vi "Main2.vi"() -> ()   [LabVIEW 2014]
uses:
  Control/Control_process.ctl
  Program Files (x86)/National Instruments/LabVIEW 2018/instr.lib/OSICS 1.1.0/OSICS_LIB.lvlib
  <vilib>/Utility/file.llb/Write Delimited Spreadsheet (string).vi
panel:
  out "EXFO_OPC 2":bool
  out "EXFO_OPC":bool
  in  "myFname":bool caption="Naming Log"
  out "error IO":errorcluster
  out "Test_pts_array":dbl[](array[numeric])
  out "WL_now":dbl
  in  "stop":bool
  in  "WL_delay(ms)":u32=200
  in  "VISA_PWM":refnum<visa-resource-name> caption="Power Meter"
  in  "VISA_TLS":refnum<visa-resource-name> caption="Light Source"
  in  "PM_delay(ms)":i32=100
  out "Ref dbm":dbl caption="Ref (dBm)" format="%#.2g"
  in  "WL_Set":dbl=1310.0 caption="Wavelength"
  out "pow_read":dbl caption="Pow" format="%#.2g"
  in  "WL_step":dbl=1.0 caption="Step(nm)"
  out "WL_Peak":dbl caption="Peak"
  in  "WL_End":dbl=1350.0 caption="End(nm)"
  in  "WL_Start":dbl=1260.0 caption="Start(nm)"
  in  "Link Button":bool
  in  "Unit(dB:T)":bool
  in  "Read Button":bool
  in  "Ref Button":bool
  in  "Ref_spec Button":bool
  out "REF?":bool caption="Ref.1pt"
  out "testing?":bool caption="Busy"
  out "link?":bool caption="Online"
  out "Msg":string
  in  "Sweep Button":bool
  out "pow_chart":dbl(graph)
  # "切換波長有OPC?指令應該是會等待執行完成的flag回傳\n不須另外放delay, 目前有家只是為了確保"
  # "不紀錄取單點參考值的波長，全波長才記\n要考慮一下做了什麼動作就清掉全波長參考值"
  # "Equip."
  # "SWEEP"
  # "READ"
  # "Ver. B01.0"
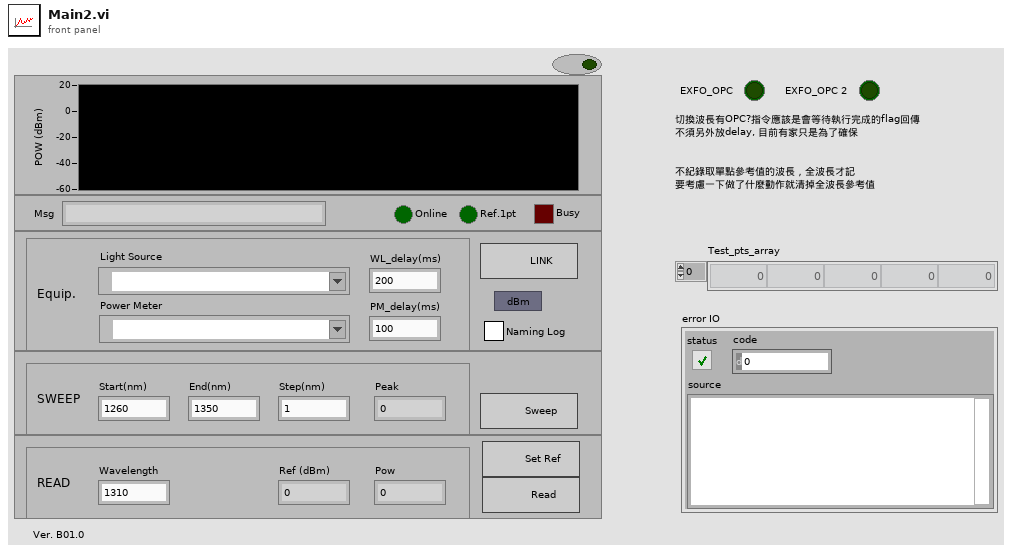
[diagram p1: front panel]
types:
  T1 = typedef "Control_process.ctl" = enum16{"init", "link", "reference", "reference2", "wave_chng", "lockpanel", "single", "sweep", "log_res", "quit"}
  T2 = enum8{"Enabled", "Disabled", "Disabled and Grayed Out"}
  T3 = cluster{"Laser State":bool, "WL/F Value":dbl, "Power (dBm/mW)":dbl, "Power Limit":bool}
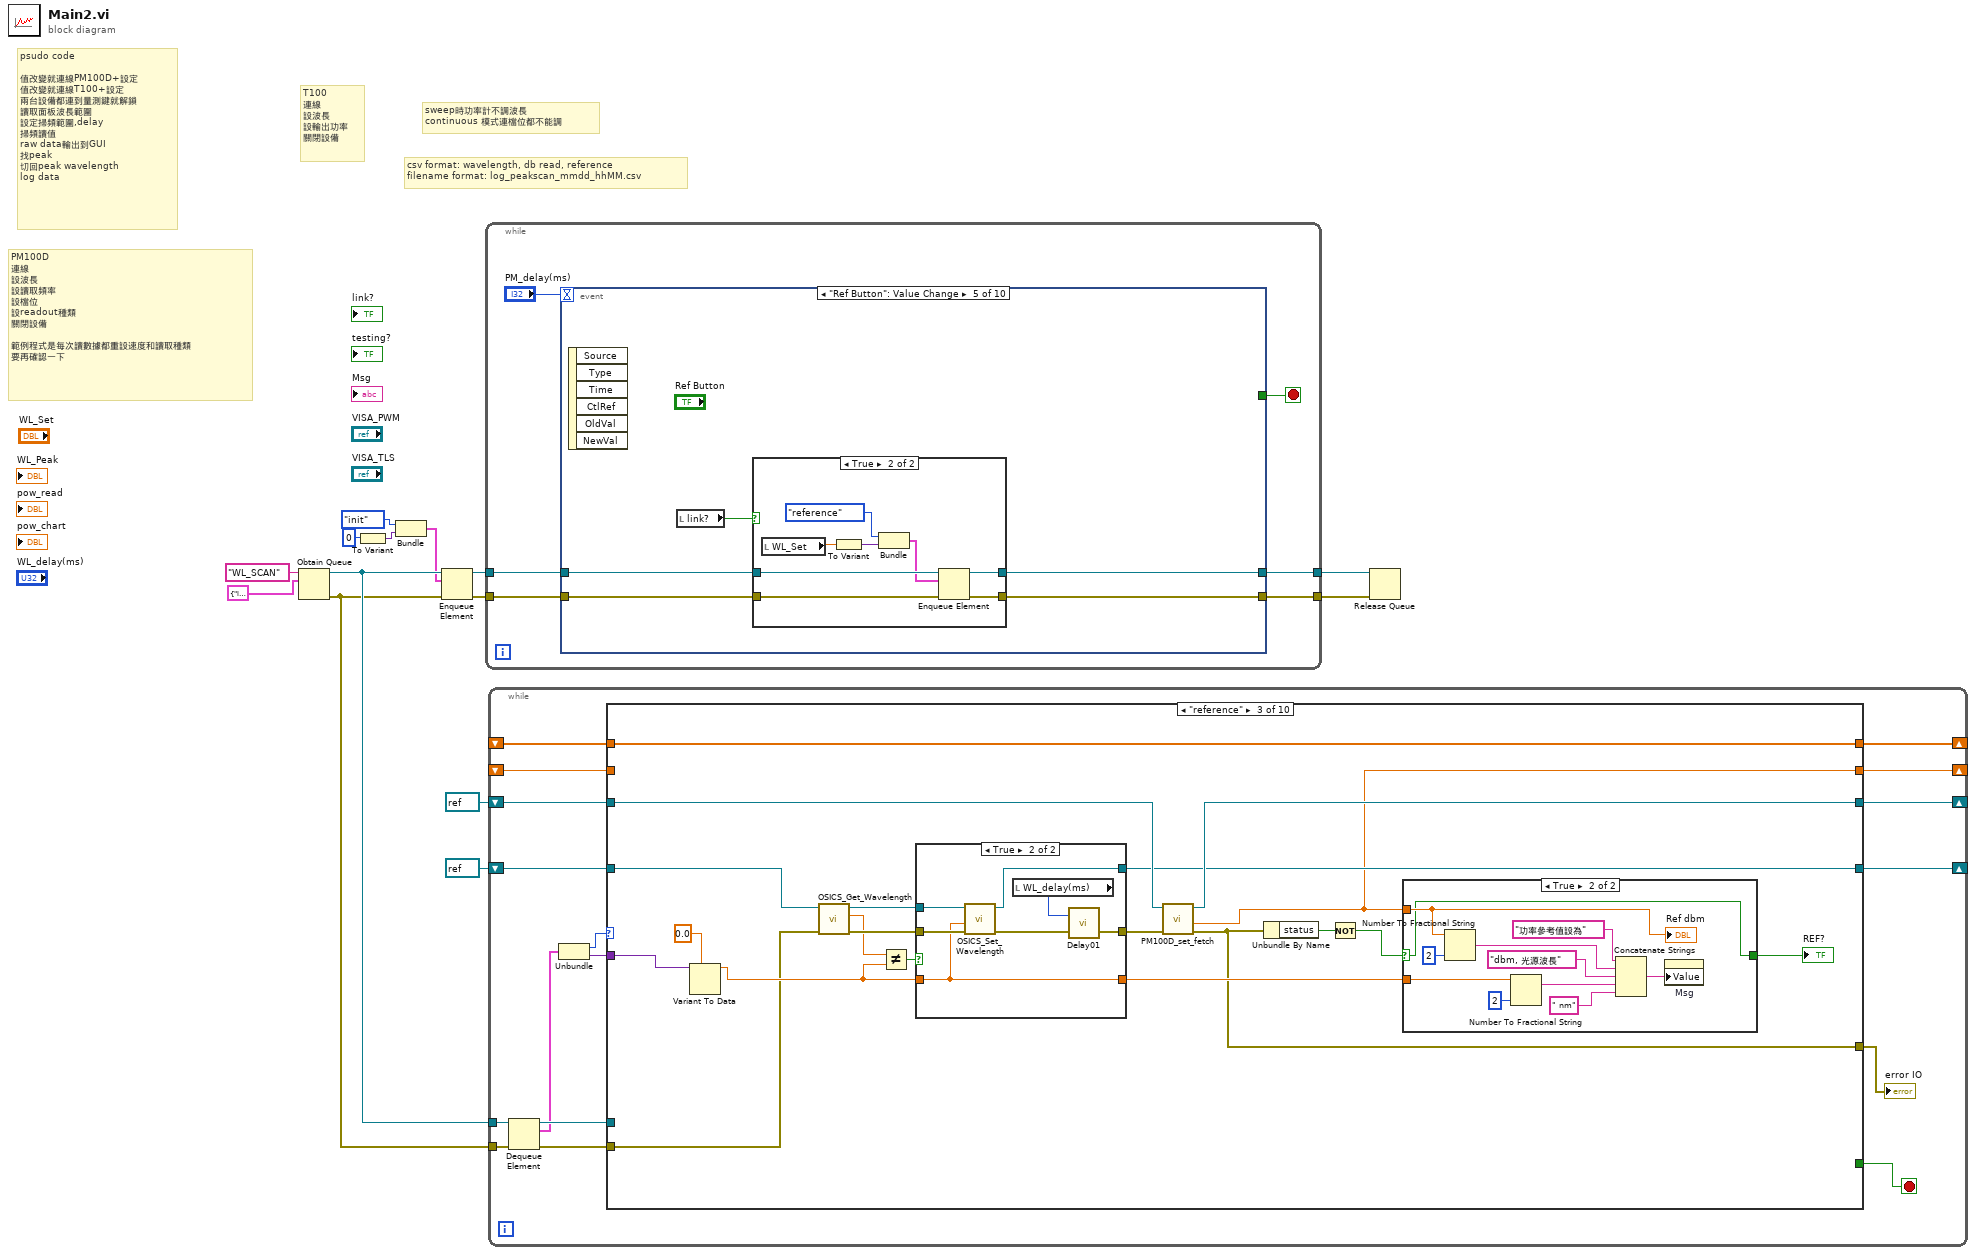
[diagram p0: block diagram]
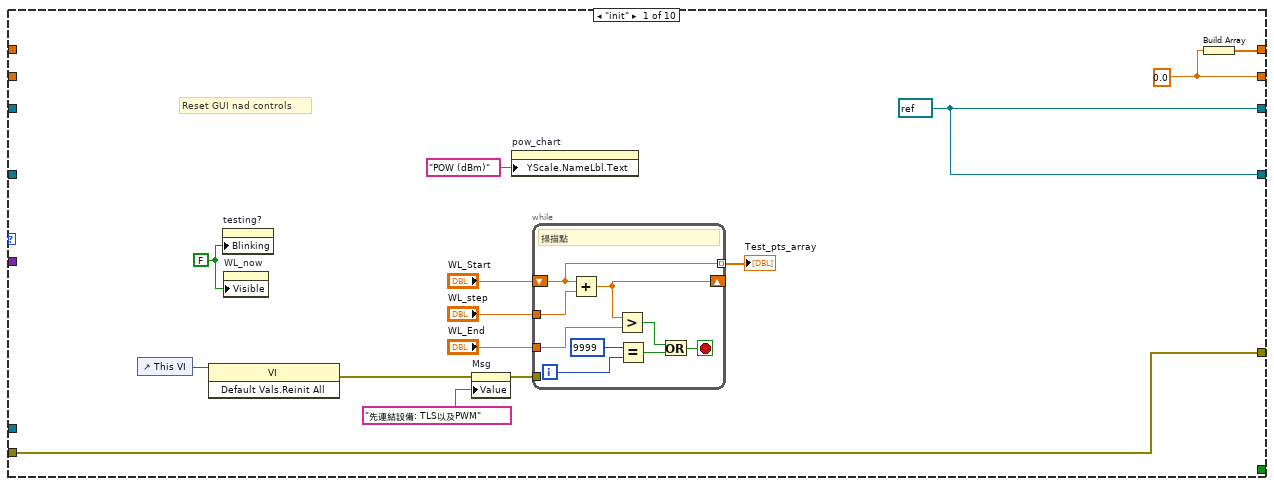
[diagram p2: hidden frame]
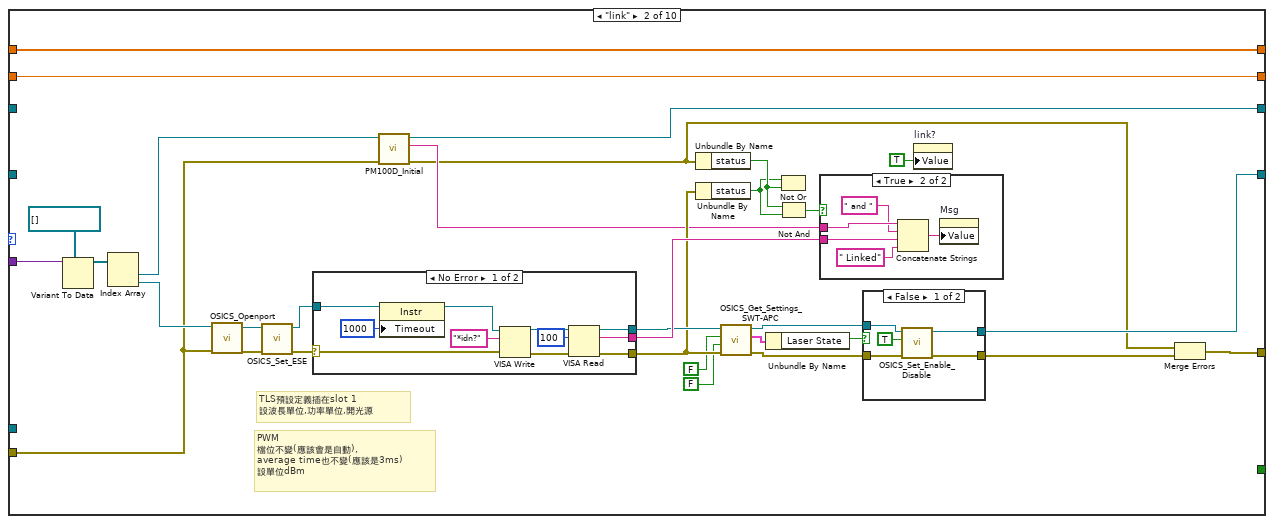
[diagram p3: hidden frame]
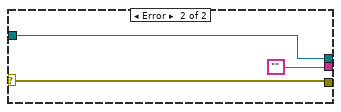
[diagram p4: hidden frame]
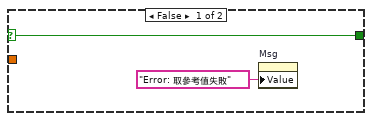
[diagram p7: hidden frame]
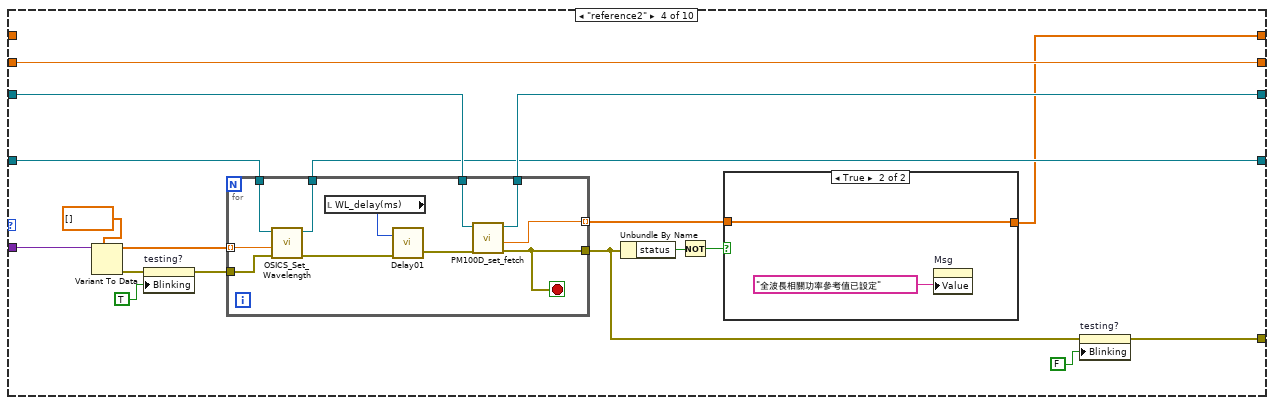
[diagram p9: hidden frame]
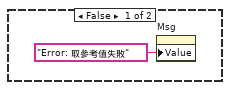
[diagram p10: hidden frame]
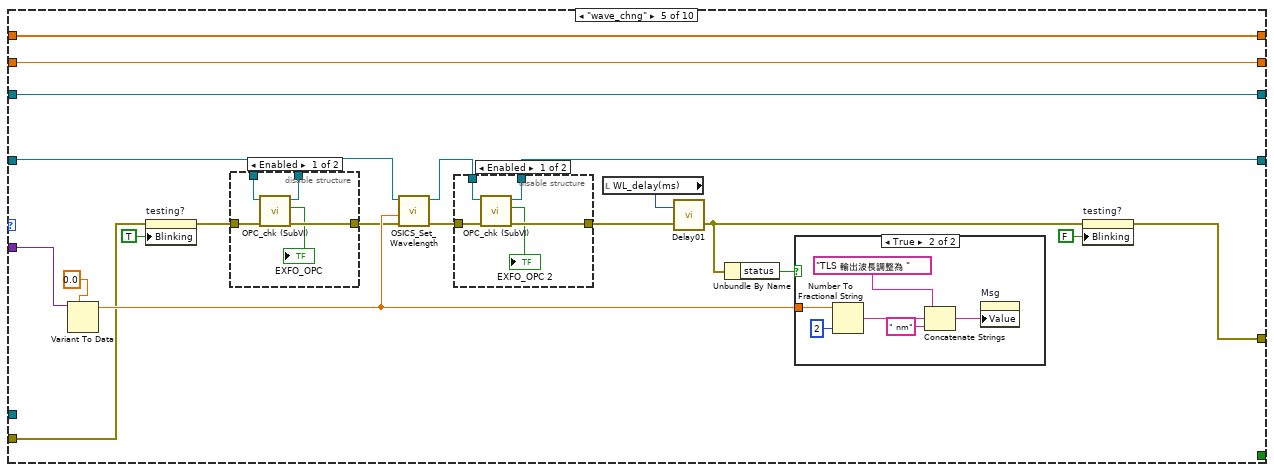
[diagram p11: hidden frame]
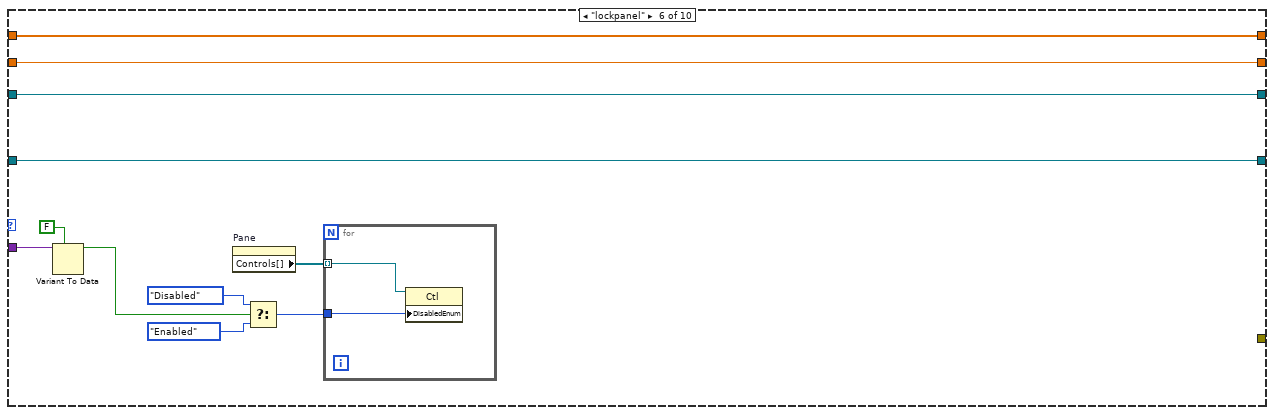
[diagram p15: hidden frame]
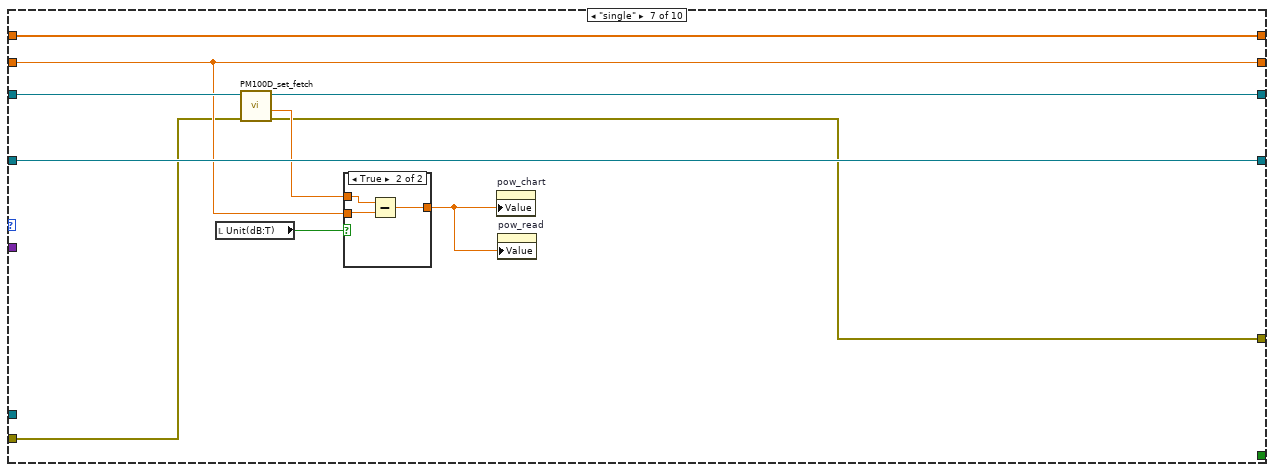
[diagram p16: hidden frame]
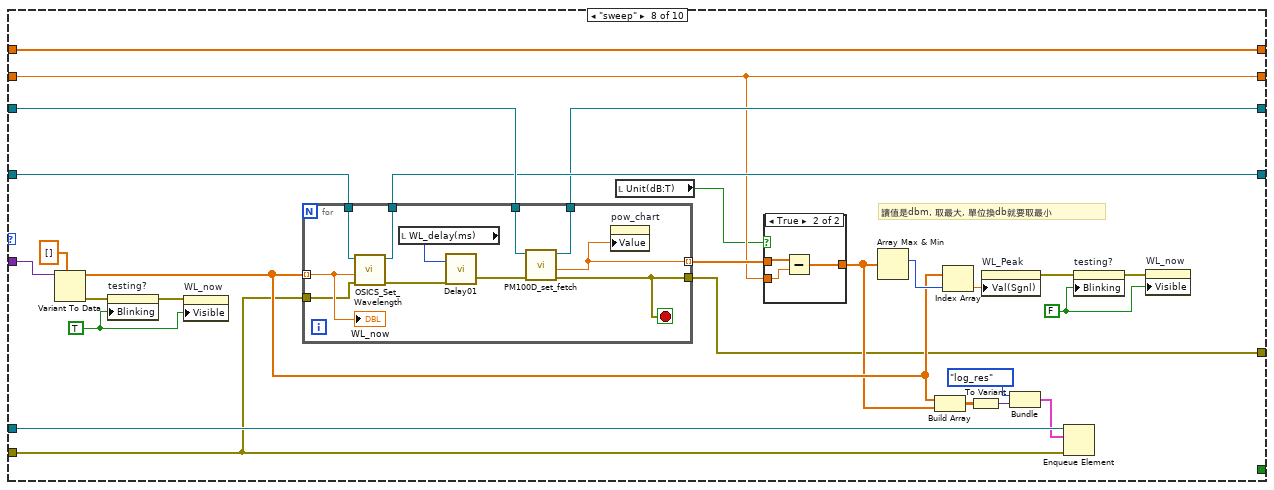
[diagram p18: hidden frame]
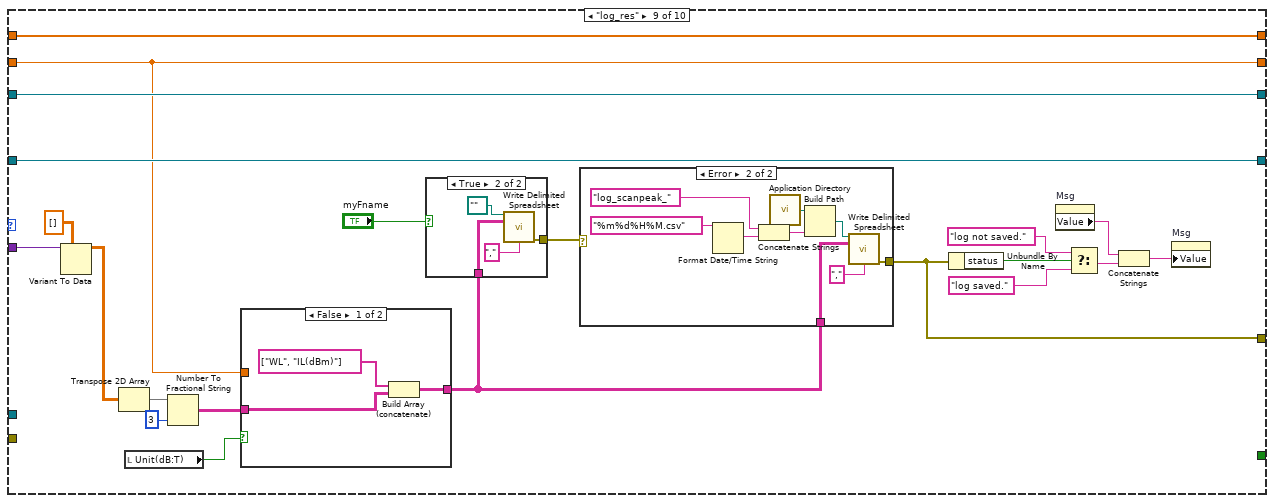
[diagram p20: hidden frame]
diagram:
  # "csv format: wavelength, db read, reference\nfilename format: log_peakscan_mmdd_hhMM.csv"
  # "sweep時功率計不調波長\ncontinuous 模式連檔位都不能調"
  # "T100\n連線\n設波長\n設輸出功率\n關閉設備"
  # "PM100D\n連線\n設波長\n設讀取頻率\n設檔位\n設readout種類\n關閉設備\n\n範例程式是每次讀數據都重設速度和讀取種類\n要再確認一下"
  # "psudo code\n\n值改變就連線PM100D+設定\n值改變就連線T100+設定\n兩台設備都連到量測鍵就解鎖\n讀取面板波長範圍\n設定掃頻範圍,delay\n掃頻讀值\nraw data輸出到GUI\n找peak\n切回peak wavelength\nlog data"
  n1 = Obtain Queue(name (unnamed)="WL_SCAN", element data type=cluster{"Proc":T1, variant} {"Proc"=enum."init", variant}) -> (queue out=w13:refnum<queue>, error out=w1:errorcluster)  [unwired: 3 in, 1 out]
  n2 = To Variant(anything=0) -> (Variant=w6:variant)
  n3 = Bundle("Proc"=Control_process."init", "Variant"=w6) -> (w4:cluster{"Proc":T1, "Variant":variant})  [unwired: 1 in]
  n4 = Enqueue Element(queue=w13, element=w4, error in (no error)=w1) -> (queue out=w9:refnum<queue>, error out=w8:errorcluster)  [unwired: 1 in, 1 out]
  n5 = while {
    tunnel: w9 -> [w18]
    tunnel: w8 -> [w19]
    tunnel: [w17] -> w12
    tunnel: [w16] -> w11
    stop <- w20 stop-if-true
    n6 = event shown="[4] \"Ref Button\": Value Change" {
      selector: _ -> [_ _ _ _ _ _ _ _ _ _]
      dyn-events: _ -> [_ _ _ _ _ _ _ _ _ _]
      timeout: "PM_delay(ms)" -> [_ _ _ _ _ _ _ _ _ _]
      tunnel: [_ _ _ _ _ _ _ _ _ TRUE] -> w20
      tunnel: w19 -> [w26 w40 w53 w75 w89 w105 w136 w146 w174 w196]
      tunnel: w18 -> [w27 w41 w54 w76 w90 w106 w132 w148 w177 w194]
      tunnel: [w25 w41 w52 w76 w88 w104 w131 w147 w176 w193] -> w17
      tunnel: [w24 w40 w51 w75 w87 w103 w136 w145 w175 w195] -> w16
      event Timeout {
        n7 = event-data() -> ()  [unwired: 1 in, 3 out]
        n8 = local read "link?"() -> (w21:bool)
        n9 = local read "Read Button"() -> (w22:bool)
        n10 = And(x=w21, y=w22) -> (x .and. y?=w23:bool)
        n11 = case shown="False" w23 {
          tunnel: w27 -> [w29 w37]
          tunnel: w26 -> [w28 w36]
          tunnel: [w29 w35] -> w25
          tunnel: [w28 w34] -> w24
          frame False {
          }
          frame True {
            n12 = To Variant(anything=0) -> (Variant=w33:variant)
            n13 = Bundle("Proc"=Control_process."single", "Variant"=w33) -> (w31:cluster{"Proc":T1, "Variant":variant})  [unwired: 1 in]
            n14 = Enqueue Element(queue=w37, element=w31, error in (no error)=w36) -> (queue out=w35:refnum<queue>, error out=w34:errorcluster)  [unwired: 1 in, 1 out]
          }
        }
      }
      event "Unit(dB:T)": Value Change {
        # "這個事件會卡有紀錄參考值才能把單位轉dB"
        n15 = event-data() -> ()  [unwired: 1 in, 6 out]
        n16 = local read "REF?"() -> (w39:bool)
        n17 = case shown="True" w39 {
          tunnel: "Unit(dB:T)" -> [_ w47]
          frame False {
            n18 = property on="Unit(dB:T)" class="Bool (strict)"("Value"=FALSE ("Unit")) -> ()  [unwired: 2 in, 2 out]
            n19 = property on="Msg" class="Str"("Value"="Error: 參考值未設定" ("Msg")) -> ()  [unwired: 2 in, 2 out]
          }
          frame True {
            n20 = Select(t="POW (dB)", s=w47, f="POW (dBm)") -> (s? t:f=w48:string)
            n21 = property on="pow_chart" class="WFChart (strict)"("YScale.NameLbl.Text"=w48, "History Data"=dbl[] []) -> ()  [unwired: 2 in, 2 out]
          }
        }
      }
      event "Link Button": Value Change {
        n22 = event-data() -> ()  [unwired: 1 in, 1 out]
        n23 = local read "VISA_PWM"() -> (w49:refnum<visa-resource-name>)
        n24 = local read "VISA_TLS"() -> (w50:refnum<visa-resource-name>)
        n25 = Empty String/Path?(string/path=w50) -> (empty?=w56:bool)
        n26 = Empty String/Path?(string/path=w49) -> (empty?=w57:bool)
        n27 = Not Or(1:w56, 2:w57) -> (0:w55:bool)
        n28 = case shown="True" w55 {
          tunnel: w54 -> [w60 w70]
          tunnel: w53 -> [w59 w69]
          tunnel: [w60 w68] -> w52
          tunnel: [w59 w67] -> w51
          tunnel: w49 -> [_ w64]
          tunnel: w50 -> [_ w63]
          frame False {
            n29 = property on="Msg" class="Str"("Value"="Error: 未選擇儀器位址" ("Msg")) -> ()  [unwired: 2 in, 2 out]
          }
          frame True {
            n30 = Build Array(w64, w63) -> (w62:refnum<visa-resource-name>[])
            n31 = To Variant(anything=w62) -> (Variant=w61:variant)
            n32 = Bundle("Proc"=Control_process."link", "Variant"=w61) -> (w65:cluster{"Proc":T1, "Variant":variant})  [unwired: 1 in]
            n33 = Enqueue Element(queue=w70, element=w65, error in (no error)=w69) -> (queue out=w68:refnum<queue>, error out=w67:errorcluster)  [unwired: 1 in, 1 out]
          }
        }
      }
      event "WL_Start", "WL_End", "WL_step": Value Change {
        n34 = event-data() -> ()  [unwired: 1 in, 6 out]
        n35 = local read "WL_Start"() -> (w72:dbl)
        n36 = local read "WL_step"() -> (w74:dbl)
        n37 = local read "WL_End"() -> (w73:dbl)
        n38 = while {
          tunnel: w74 -> [w80]
          tunnel: w73 -> [w79]
          shift-right: [w81] -> _
          shift-left: w72 -> [w82]
          tunnel: [w82] -> w71 mode=indexing
          i -> [w78]
          stop <- w77 stop-if-true
          # "掃描點"
          n39 = Add(x=w82, y=w80) -> (x+y=w81:dbl)
          n40 = Greater?(x=w81, y=w79) -> (0:w84:bool)
          n41 = Equal?(x=9999, y=w78) -> (x = y?=w83:bool)
          n42 = Or(x=w84, y=w83) -> (x .or. y?=w77:bool)
        }
        n43 = local write "Test_pts_array"(w71) -> ()
      }
      event "Ref Button": Value Change {
        n44 = event-data() -> ()  [unwired: 1 in, 6 out]
        n45 = local read "link?"() -> (w86:bool)
        n46 = case shown="True" w86 {
          tunnel: w90 -> [w93 w101]
          tunnel: w89 -> [w92 w100]
          tunnel: [w93 w99] -> w88
          tunnel: [w92 w98] -> w87
          frame False {
            n47 = property on="Msg" class="Str"("Value"="Err: 設備未連結" ("Msg")) -> ()  [unwired: 2 in, 2 out]
          }
          frame True {
            n48 = local read "WL_Set"() -> (w94:dbl)
            n49 = To Variant(anything=w94) -> (Variant=w97:variant)
            n50 = Bundle("Proc"=Control_process."reference", "Variant"=w97) -> (w95:cluster{"Proc":T1, "Variant":variant})  [unwired: 1 in]
            n51 = Enqueue Element(queue=w101, element=w95, error in (no error)=w100) -> (queue out=w99:refnum<queue>, error out=w98:errorcluster)  [unwired: 1 in, 1 out]
          }
        }
      }
      event "Ref_spec Button": Value Change {
        n52 = event-data() -> ()  [unwired: 1 in, 6 out]
        n53 = local read "link?"() -> (w102:bool)
        n54 = case shown="True" w102 {
          tunnel: w106 -> [w109 w117]
          tunnel: w105 -> [w108 w116]
          tunnel: [w109 w113] -> w104
          tunnel: [w108 w110] -> w103
          frame False {
            n55 = property on="Msg" class="Str"("Value"="Error: 設備未連結" ("Msg")) -> ()  [unwired: 2 in, 2 out]
          }
          frame True {
            n56 = To Variant(anything=TRUE) -> (Variant=w123:variant)
            n57 = Bundle("Proc"=Control_process."lockpanel", "Variant"=w123) -> (w125:cluster{"Proc":T1, "Variant":variant})  [unwired: 1 in]
            n58 = local read "WL_Set"() -> (w126:dbl)
            n59 = Enqueue Element(queue=w117, element=w125, error in (no error)=w116) -> (queue out=w111:refnum<queue>, error out=w115:errorcluster)  [unwired: 1 in, 1 out]
            n60 = To Variant(anything=w126) -> (Variant=w129:variant)
            n61 = Bundle("Proc"=Control_process."reference", "Variant"=w129) -> (w127:cluster{"Proc":T1, "Variant":variant})  [unwired: 1 in]
            n62 = Enqueue Element(queue=w111, element=w127, error in (no error)=w115) -> (queue out=w112:refnum<queue>, error out=w114:errorcluster)  [unwired: 1 in, 1 out]
            n63 = To Variant(anything=FALSE) -> (Variant=w120:variant)
            n64 = Bundle("Proc"=Control_process."lockpanel", "Variant"=w120) -> (w118:cluster{"Proc":T1, "Variant":variant})  [unwired: 1 in]
            n65 = Enqueue Element(queue=w112, element=w118, error in (no error)=w114) -> (queue out=w113:refnum<queue>, error out=w110:errorcluster)  [unwired: 1 in, 1 out]
          }
        }
      }
      event "Read Button": Value Change {
        n66 = event-data() -> ()  [unwired: 1 in, 6 out]
        n67 = local read "link?"() -> (w134:bool)
        n68 = And(x=w134, y="Read Button") -> (x .and. y?=w133:bool)
        n69 = case shown="False" w133 {
          selector: w133 -> [w141 w142]
          tunnel: w132 -> [w139 w143]
          tunnel: [w138 w143] -> w131
          tunnel: [FALSE ("Blinking") w142] -> w130
          frame False {
            n70 = property on="Read Button" class="Bool (strict)"("Value"=w141) -> ()  [unwired: 2 in, 2 out]
            n71 = property on="Msg" class="Str"("Value"="Error: 設備未連結" ("Msg")) -> ()  [unwired: 2 in, 2 out]
            n72 = Flush Queue(queue=w139) -> (queue out=w138:refnum<queue>)  [unwired: 1 in, 2 out]
          }
          frame True {
          }
        }
        n73 = property on="testing?" class="Bool (strict)"("Blinking"=w130) -> ()  [unwired: 2 in, 2 out]
      }
      event "Sweep Button": Value Change {
        n74 = event-data() -> ()  [unwired: 1 in, 1 out]
        n75 = local read "link?"() -> (w144:bool)
        n76 = case shown="True" w144 {
          tunnel: w148 -> [w151 w155]
          tunnel: [w151 w161] -> w147
          tunnel: w146 -> [w150 w159]
          tunnel: [w150 w156] -> w145
          frame False {
            n77 = property on="Msg" class="Str"("Value"="Err: 設備未連結" ("Msg")) -> ()  [unwired: 2 in, 2 out]
          }
          frame True {
            n78 = To Variant(anything=TRUE) -> (Variant=w167:variant)
            n79 = Bundle("Proc"=Control_process."lockpanel", "Variant"=w167) -> (w168:cluster{"Proc":T1, "Variant":variant})  [unwired: 1 in]
            n80 = local read "Test_pts_array"() -> (w152:dbl[])
            n81 = Enqueue Element(queue=w155, element=w168, error in (no error)=w159) -> (queue out=w154:refnum<queue>, error out=w158:errorcluster)  [unwired: 1 in, 1 out]
            n82 = To Variant(anything=w152) -> (Variant=w171:variant)
            n83 = Bundle("Proc"=Control_process."sweep", "Variant"=w171) -> (w170:cluster{"Proc":T1, "Variant":variant})  [unwired: 1 in]
            n84 = Enqueue Element(queue=w154, element=w170, error in (no error)=w158) -> (queue out=w153:refnum<queue>, error out=w157:errorcluster)  [unwired: 1 in, 1 out]
            n85 = To Variant(anything=FALSE) -> (Variant=w164:variant)
            n86 = Bundle("Proc"=Control_process."lockpanel", "Variant"=w164) -> (w163:cluster{"Proc":T1, "Variant":variant})  [unwired: 1 in]
            n87 = Enqueue Element(queue=w153, element=w163, error in (no error)=w157) -> (queue out=w161:refnum<queue>, error out=w156:errorcluster)  [unwired: 1 in, 1 out]
            n88 = property on="Msg" class="Str"("Value"="波長掃描中......" ("Msg")) -> ()  [unwired: 2 in, 2 out]
          }
        }
      }
      event "WL_Set", "WL_Peak": Value Change {
        n89 = event-data() -> ("NewVal"=w178:dbl)  [unwired: 1 in]
        n90 = local read "link?"() -> (w173:bool)
        n91 = case shown="True" w173 {
          tunnel: w178 -> [_ w187]
          tunnel: w177 -> [w180 w185]
          tunnel: [w180 w184] -> w176
          tunnel: [w179 w183] -> w175
          tunnel: w174 -> [w179 w182]
          frame False {
          }
          frame True {
            n92 = To Variant(anything=w187) -> (Variant=w188:variant)
            n93 = Bundle("Proc"=Control_process."wave_chng", "Variant"=w188) -> (w181:cluster{"Proc":T1, "Variant":variant})  [unwired: 1 in]
            n94 = Enqueue Element(queue=w185, element=w181, error in (no error)=w182) -> (queue out=w184:refnum<queue>, error out=w183:errorcluster)  [unwired: 1 in, 1 out]
          }
        }
      }
      event "stop": Value Change {
        n95 = event-data() -> ()  [unwired: 1 in, 6 out]
        n96 = local read "link?"() -> (w189:bool)
        n97 = To Variant(anything=w189) -> (Variant=w191:variant)
        n98 = Bundle("Proc"=Control_process."quit", "Variant"=w191) -> (w190:cluster{"Proc":T1, "Variant":variant})  [unwired: 1 in]
        n99 = Enqueue Element At Opposite End(queue=w194, element=w190, error in (no error)=w196) -> (queue out=w193:refnum<queue>, error out=w195:errorcluster)  [unwired: 1 in, 1 out]
      }
    }
  }
  n100 = while {
    tunnel: w13 -> [w214]
    shift-right: [w204] -> _
    shift-left: refnum<visa-resource-name> refnum ("instrument handle out") -> [w208]
    shift-right: [w207] -> _
    shift-left: refnum<visa-resource-name> refnum ("VISA OUT") -> [w206]
    shift-right: [w203] -> _
    shift-left: _ -> [w202]
    tunnel: w1 -> [w200]
    shift-right: [w198] -> _
    shift-left: _ -> [w199]
    stop <- w205 stop-if-true
    n101 = Dequeue Element(queue=w214, error in (no error)=w200) -> (queue out=w213:refnum<queue>, element=w211:cluster{"Proc":T1, variant}, error out=w212:errorcluster)  [unwired: 1 in, 1 out]
    n102 = Unbundle(w211) -> ("Proc"=w210:T1, w209:variant)
    n103 = case shown="\"reference\"" w210 {
      tunnel: w213 -> [_ _ _ _ _ _ _ w456 _ _]
      tunnel: w212 -> [w226 w239 w302 _ w379 _ w425 w439 _ w529]
      tunnel: w209 -> [_ w268 w312 w355 w390 w414 _ w463 w499 w533]
      tunnel: w208 -> [_ _ w314 w350 w386 w420 w433 w464 w491 w536]
      tunnel: [w228 w252 w311 w348 w372 w419 w432 w462 w498 w534] -> w207
      tunnel: w206 -> [_ _ w309 w351 w374 w419 w432 w461 w498 w538]
      tunnel: [_ _ _ _ _ _ _ _ _ TRUE] -> w205
      tunnel: [w228 w244 w313 w349 w386 w420 w431 w451 w491 w535] -> w204
      tunnel: [w226 w248 w301 w344 w382 _ w426 w446 w486 w528] -> w201
      tunnel: [w219 w249 w298 w352 w384 w421 w429 w449 w485 w530] -> w203
      tunnel: w202 -> [_ w249 _ w352 w384 w421 w429 w449 w485 w530]
      tunnel: w199 -> [_ w238 w295 _ w370 w411 w424 w438 w480 w526]
      tunnel: [w218 w238 w295 w339 w370 w411 w424 w438 w480 w526] -> w198
      frame "init" {
        w219 = 0.0
        w225 = FALSE ("Blinking")
        w228 = refnum<visa-resource-name> refnum ("instrument handle out")
        # "Reset GUI nad controls"
        n104 = control-ref of="This VI"() -> (w227:refnum<vi>)
        n105 = invoke class="VI" method="Default Vals.Reinit All"(reference=w227) -> (error out=w216:errorcluster)  [unwired: 2 in, 2 out]
        n106 = property on="testing?" class="Bool (strict)"("Blinking"=w225) -> ()  [unwired: 2 in, 2 out]
        n107 = property on="WL_now" class="DigNum (strict)"("Visible"=w225) -> ()  [unwired: 2 in, 2 out]
        n108 = property on="Msg" class="Str"(error in=w216, "Value"="先連結設備: TLS以及PWM" ("string")) -> (error out=w215:errorcluster)  [unwired: 1 in, 1 out]
        n109 = property on="pow_chart" class="WFChart (strict)"("YScale.NameLbl.Text"="POW (dBm)") -> ()  [unwired: 2 in, 2 out]
        n110 = while {
          tunnel: "WL_step" -> [w232]
          tunnel: "WL_End" -> [w231]
          shift-right: [w233] -> _
          shift-left: "WL_Start" -> [w234]
          tunnel: [w234] -> w221 mode=indexing
          tunnel: w215 -> [_]
          i -> [w230]
          stop <- w229 stop-if-true
          # "掃描點"
          n111 = Add(x=w234, y=w232) -> (x+y=w233:dbl)
          n112 = Greater?(x=w233, y=w231) -> (0:w236:bool)
          n113 = Equal?(x=9999, y=w230) -> (x = y?=w235:bool)
          n114 = Or(x=w236, y=w235) -> (x .or. y?=w229:bool)
        }
        "Test_pts_array" <- w221
        n115 = Build Array(w219) -> (w218:dbl[])
      }
      frame "link" {
        # "TLS預設定義插在slot 1\n設波長單位,功率單位,開光源"
        # "PWM\n檔位不變(應該會是自動), \naverage time也不變(應該是3ms)\n設單位dBm"
        n116 = Variant To Data(type=refnum<visa-resource-name>[] [], Variant=w268) -> (data=w267:refnum<visa-resource-name>[])  [unwired: 1 in, 1 out]
        n117 = Index Array(array=w267) -> (element #1=w245:refnum<visa-resource-name>, element #2=w265:refnum<visa-resource-name>)  [unwired: 2 in]
        n118 = call "OSICS_Openport.vi"("error in"=w239, "VISA IN"=w265) -> ("error out"=w266:errorcluster, "VISA OUT"=w264:refnum<visa-resource-name>)  [unwired: 8 in]
        n119 = call "OSICS_Set_ESE.vi"("error in (no error)"=w266, "VISA resource name"=w264) -> ("error out"=w242:errorcluster, "VISA resource name out"=w263:refnum<visa-resource-name>)  [unwired: 8 in]
        n120 = case shown="No Error" w242 {
          selector: w242 -> [w269 w282]
          tunnel: w263 -> [w273 w281]
          tunnel: [w272 ""] -> w262
          tunnel: [w271 w281] -> w260
          tunnel: [w270 w282] -> w257
          frame No Error {
            n121 = property class="Instr"(reference=w273, "Timeout"=u32 1000 ("General Settings:Timeout Value")) -> (reference out=w278:refnum<visa-resource-name>)  [unwired: 1 in, 1 out]
            n122 = VISA Write(VISA resource name=w278, write buffer="*idn?", error in (no error)=w269) -> (VISA resource name out=w276:refnum<visa-resource-name>, error out=w274:errorcluster)  [unwired: 1 out]
            n123 = VISA Read(VISA resource name=w276, byte count=u32 100, error in (no error)=w274) -> (VISA resource name out=w271:refnum<visa-resource-name>, read buffer=w272:string, error out=w270:errorcluster)  [unwired: 1 out]
          }
          frame Error {
          }
        }
        n124 = call "PM100D_Initial.vi"("error in"=w239, "VISA in"=w245) -> ("error out"=w243:errorcluster, "IDN String"=w246:string, "VISA out"=w244:refnum<visa-resource-name>)  [unwired: 2 in, 1 out]
        n125 = Unbundle By Name(w243) -> ("status"=w251:bool)
        n126 = Unbundle By Name(w257) -> ("status"=w250:bool)
        n127 = call "OSICS_Get_Settings_SWT-APC.vi"("error in"=w257, "Power Unit(dBm/mW)"=FALSE, "WL/F unit (nm/GHz)"=FALSE, "VISA IN"=w260) -> ("error out"=w253:errorcluster, "Laser Settings (Cluster)"=w259:T3, "VISA OUT"=w254:refnum<visa-resource-name>)  [unwired: 5 in]
        n128 = Unbundle By Name(w259) -> ("Laser State"=w258:bool)
        n129 = Not Or(1:w251, 2:w250) -> ()  [unwired: 1 out]
        n130 = Not And(1:w250, 2:w251) -> (0:w261:bool)
        n131 = case shown="True" w261 {
          tunnel: w262 -> [_ w294]
          tunnel: w246 -> [_ w293]
          frame False {
          }
          frame True {
            n132 = Concatenate Strings(w293, " and " ("string"), w294, " Linked" ("string")) -> (w291:string)
            n133 = property on="Msg" class="Str"("Value"=w291) -> ()  [unwired: 2 in, 2 out]
          }
        }
        n134 = case shown="False" w258 {
          tunnel: w254 -> [w286 w289]
          tunnel: w253 -> [w285 w288]
          tunnel: [w284 w289] -> w252
          tunnel: [w283 w288] -> w240
          frame False {
            n135 = call "OSICS_Set_Enable_Disable.vi"("error in"=w285, "Laser State (False:DISABLED)"=TRUE, "VISA IN"=w286) -> ("error out"=w283:errorcluster, "VISA OUT"=w284:refnum<visa-resource-name>)  [unwired: 6 in, 1 out]
          }
          frame True {
          }
        }
        n136 = property on="link?" class="Bool (strict)"("Value"=TRUE ("link?")) -> ()  [unwired: 2 in, 2 out]
        n137 = Merge Errors(w243, w240) -> (w248:errorcluster)
      }
      frame "reference" {
        n138 = Variant To Data(type=0.0, Variant=w312) -> (data=w303:dbl)  [unwired: 1 in, 1 out]
        n139 = call "OSICS_Get_Wavelength.vi"("error in"=w302, "VISA IN"=w309) -> ("error out"=w308:errorcluster, "WL/Frequency Value"=w306:dbl, "VISA OUT"=w310:refnum<visa-resource-name>)  [unwired: 6 in, 1 out]
        n140 = Not Equal?(x=w306, y=w303) -> (x != y?=w307:bool)
        n141 = case shown="True" w307 {
          tunnel: [w329 w335] -> w299
          tunnel: [w330 w334] -> w311
          tunnel: w310 -> [w330 w333]
          tunnel: w308 -> [w329 w332]
          tunnel: w303 -> [w328 w331]
          tunnel: [w328 w331] -> w305
          frame False {
          }
          frame True {
            n142 = call "OSICS_Set_Wavelength.vi"("error in"=w332, "WL/Frequency Value"=w331, "VISA IN"=w333) -> ("error out"=w337:errorcluster, "VISA OUT"=w334:refnum<visa-resource-name>)  [unwired: 6 in, 1 out]
            n143 = local read "WL_delay(ms)"() -> (w336:u32)
            n144 = call "Delay01.vi"("error in"=w337, "ms delay"=w336) -> ("error out"=w335:errorcluster)  [unwired: 1 in]
          }
        }
        n145 = call "PM100D_set_fetch.vi"("error in"=w299, "VISA in"=w314) -> ("error out"=w301:errorcluster, "Readout value"=w298:dbl, "VISA out"=w313:refnum<visa-resource-name>)  [unwired: 5 in, 2 out]
        n146 = Unbundle By Name(w301) -> ("status"=w300:bool)
        n147 = Not(x=w300) -> (.not. x?=w297:bool)
        n148 = case shown="True" w297 {
          selector: w297 -> [w316 w317]
          tunnel: w305 -> [_ w319]
          tunnel: w298 -> [_ w318]
          tunnel: [w316 w317] -> w296
          frame False {
            n149 = property on="Msg" class="Str"("Value"="Error: 取參考值失敗" ("Msg")) -> ()  [unwired: 2 in, 2 out]
          }
          frame True {
            n150 = Number To Fractional String(number=w318, precision (6)=i16 2) -> (F-format string=w321:string)  [unwired: 2 in]
            n151 = Number To Fractional String(number=w319, precision (6)=i16 2) -> (F-format string=w325:string)  [unwired: 2 in]
            n152 = Concatenate Strings("功率參考值設為" ("string"), w321, "dbm, 光源波長" ("string"), w325, " nm" ("string")) -> (w324:string)
            n153 = property on="Msg" class="Str"("Value"=w324) -> ()  [unwired: 2 in, 2 out]
            "Ref dbm" <- w318
          }
        }
        "REF?" <- w296
      }
      frame "reference2" {
        n154 = Variant To Data(type=dbl[] [], Variant=w355) -> (data=w353:dbl[], error out=w345:errorcluster)  [unwired: 1 in]
        n155 = property on="testing?" class="Bool (strict)"(error in=w345, "Blinking"=TRUE) -> (error out=w338:errorcluster)  [unwired: 1 in, 1 out]
        n156 = for {
          tunnel: w350 -> [w369]
          tunnel: [w368] -> w349
          tunnel: [w365] -> w348
          tunnel: w351 -> [w364]
          tunnel: [w361] -> w342
          tunnel: [w363] -> w340 mode=indexing
          tunnel: w353 -> [w362] mode=indexing
          tunnel: w338 -> [w359]
          stop <- w361 stop-if-true
          n157 = call "OSICS_Set_Wavelength.vi"("error in"=w359, "WL/Frequency Value"=w362, "VISA IN"=w364) -> ("error out"=w367:errorcluster, "VISA OUT"=w365:refnum<visa-resource-name>)  [unwired: 6 in, 1 out]
          n158 = local read "WL_delay(ms)"() -> (w360:u32)
          n159 = call "Delay01.vi"("error in"=w367, "ms delay"=w360) -> ("error out"=w366:errorcluster)  [unwired: 1 in]
          n160 = call "PM100D_set_fetch.vi"("error in"=w366, "VISA in"=w369) -> ("error out"=w361:errorcluster, "Readout value"=w363:dbl, "VISA out"=w368:refnum<visa-resource-name>)  [unwired: 5 in, 2 out]
        }
        n161 = Unbundle By Name(w342) -> ("status"=w343:bool)
        n162 = Not(x=w343) -> (.not. x?=w341:bool)
        n163 = case shown="True" w341 {
          tunnel: w340 -> [_ w357]
          tunnel: [_ w357] -> w339
          frame False {
            n164 = property on="Msg" class="Str"("Value"="Error: 取參考值失敗" ("Msg")) -> ()  [unwired: 2 in, 2 out]
          }
          frame True {
            n165 = property on="Msg" class="Str"("Value"="全波長相關功率參考值已設定" ("string")) -> ()  [unwired: 2 in, 2 out]
          }
        }
        n166 = property on="testing?" class="Bool (strict)"(error in=w342, "Blinking"=FALSE) -> (error out=w344:errorcluster)  [unwired: 1 in, 1 out]
      }
      frame "wave_chng" {
        n167 = Variant To Data(type=0.0, Variant=w390) -> (data=w385:dbl)  [unwired: 1 in, 1 out]
        n168 = property on="testing?" class="Bool (strict)"(error in=w379, "Blinking"=TRUE) -> (error out=w378:errorcluster)  [unwired: 1 in, 1 out]
        n169 = disable-structure shown="Enabled" {
          disable-tunnel: w378 -> [w402 w403]
          disable-tunnel: [w401 w403] -> w375
          disable-tunnel: w374 -> [w400 w404]
          disable-tunnel: [w399 w404] -> w373
          frame Enabled {
            n170 = call "OPC_chk (SubVI).vi"("error in"=w402, "VISA in"=w400) -> ("error out"=w401:errorcluster, "opc?"=→"EXFO_OPC":bool, "VISA out"=w399:refnum<visa-resource-name>)  [unwired: 3 in]
          }
          frame Disabled {
          }
        }
        n171 = call "OSICS_Set_Wavelength.vi"("error in"=w375, "WL/Frequency Value"=w385, "VISA IN"=w373) -> ("error out"=w377:errorcluster, "VISA OUT"=w371:refnum<visa-resource-name>)  [unwired: 6 in, 1 out]
        n172 = disable-structure shown="Enabled" {
          disable-tunnel: w377 -> [w395 w396]
          disable-tunnel: [w394 w396] -> w376
          disable-tunnel: [w393 w397] -> w372
          disable-tunnel: w371 -> [w392 w397]
          frame Enabled {
            n173 = call "OPC_chk (SubVI).vi"("error in"=w395, "VISA in"=w392) -> ("error out"=w394:errorcluster, "opc?"=→"EXFO_OPC 2":bool, "VISA out"=w393:refnum<visa-resource-name>)  [unwired: 3 in]
          }
          frame Disabled {
          }
        }
        n174 = local read "WL_delay(ms)"() -> (w387:u32)
        n175 = call "Delay01.vi"("error in"=w376, "ms delay"=w387) -> ("error out"=w381:errorcluster)  [unwired: 1 in]
        n176 = Unbundle By Name(w381) -> ("status"=w388:bool)
        n177 = case shown="True" w388 {
          tunnel: w385 -> [_ w407]
          frame False {
          }
          frame True {
            n178 = Number To Fractional String(number=w407, precision (6)=i16 2) -> (F-format string=w406:string)  [unwired: 2 in]
            n179 = Concatenate Strings("TLS 輸出波長調整為 " ("Msg"), w406, " nm" ("string")) -> (w410:string)
            n180 = property on="Msg" class="Str"("Value"=w410) -> ()  [unwired: 2 in, 2 out]
          }
        }
        n181 = property on="testing?" class="Bool (strict)"(error in=w381, "Blinking"=FALSE) -> (error out=w382:errorcluster)  [unwired: 1 in, 1 out]
      }
      frame "lockpanel" {
        n182 = Variant To Data(type=FALSE, Variant=w414) -> (data=w412:bool)  [unwired: 1 in, 1 out]
        n183 = property on="Pane" class="Pane"() -> ("Controls[]"=w418:refnum<vi>[])  [unwired: 2 in, 2 out]
        n184 = Select(t=T2."Disabled" ("Disabled"), s=w412, f=T2."Enabled" ("Disabled")) -> (s? t:f=w417:T2)
        n185 = for {
          tunnel: w418 -> [w423] mode=indexing
          tunnel: w417 -> [w422]
          n186 = property on="Property Node" class="Ctl"(reference=w423, "DisabledEnum"=w422) -> ()  [unwired: 1 in, 2 out]
        }
      }
      frame "single" {
        n187 = local read "Unit(dB:T)"() -> (w427:bool)
        n188 = call "PM100D_set_fetch.vi"("error in"=w425, "VISA in"=w433) -> ("error out"=w426:errorcluster, "Readout value"=w430:dbl, "VISA out"=w431:refnum<visa-resource-name>)  [unwired: 5 in, 2 out]
        n189 = case shown="True" w427 {
          tunnel: w430 -> [w434 w437]
          tunnel: w429 -> [_ w436]
          tunnel: [w434 w435] -> w428
          frame False {
          }
          frame True {
            n190 = Subtract(x=w437, y=w436) -> (x-y=w435:dbl)
          }
        }
        n191 = property on="pow_chart" class="WFChart (strict)"("Value"=w428) -> ()  [unwired: 2 in, 2 out]
        n192 = property on="pow_read" class="DigNum (strict)"("Value"=w428) -> ()  [unwired: 2 in, 2 out]
      }
      frame "sweep" {
        w440 = TRUE ("Blinking")
        w441 = FALSE ("Blinking")
        # "讀值是dbm, 取最大, 單位換db就要取最小"
        n193 = Variant To Data(type=dbl[] [], Variant=w463) -> (data=w457:dbl[], error out=w445:errorcluster)  [unwired: 1 in]
        n194 = property on="testing?" class="Bool (strict)"(error in=w445, "Blinking"=w440) -> (error out=w443:errorcluster)  [unwired: 1 in, 1 out]
        n195 = property on="WL_now" class="DigNum (strict)"(error in=w443, "Visible"=w440) -> ()  [unwired: 1 in, 2 out]
        n196 = for {
          tunnel: w464 -> [w479]
          tunnel: [w478] -> w451
          tunnel: [w475] -> w462
          tunnel: w461 -> [w474]
          tunnel: [w471] -> w446
          tunnel: [w473] -> w450 mode=indexing
          tunnel: w457 -> [w472] mode=indexing
          tunnel: w439 -> [w469]
          stop <- w471 stop-if-true
          n197 = call "OSICS_Set_Wavelength.vi"("error in"=w469, "WL/Frequency Value"=w472, "VISA IN"=w474) -> ("error out"=w477:errorcluster, "VISA OUT"=w475:refnum<visa-resource-name>)  [unwired: 6 in, 1 out]
          n198 = local read "WL_delay(ms)"() -> (w476:u32)
          n199 = call "Delay01.vi"("error in"=w477, "ms delay"=w476) -> ("error out"=w470:errorcluster)  [unwired: 1 in]
          n200 = call "PM100D_set_fetch.vi"("error in"=w470, "VISA in"=w479) -> ("error out"=w471:errorcluster, "Readout value"=w473:dbl, "VISA out"=w478:refnum<visa-resource-name>)  [unwired: 5 in, 2 out]
          n201 = property on="pow_chart" class="WFChart (strict)"("Value"=w473) -> ()  [unwired: 2 in, 2 out]
          "WL_now" <- w472
        }
        n202 = local read "Unit(dB:T)"() -> (w447:bool)
        n203 = case shown="True" w447 {
          tunnel: w450 -> [w465 w468]
          tunnel: w449 -> [_ w467]
          tunnel: [w465 w466] -> w448
          frame False {
          }
          frame True {
            n204 = Subtract(x=w468, y=w467) -> (x-y=w466:dbl[])
          }
        }
        n205 = Array Max & Min(array=w448) -> (max index (indices)=w459:i32)  [unwired: 3 out]
        n206 = Build Array(w457, w448) -> (w453:dbl[][])
        n207 = Index Array(array=w457, index=w459) -> (element=w458:dbl)
        n208 = To Variant(anything=w453) -> (Variant=w454:variant)
        n209 = property on="WL_Peak" class="DigNum (strict)"("Val(Sgnl)"=w458) -> (error out=w444:errorcluster)  [unwired: 2 in, 1 out]
        n210 = Bundle("Proc"=Control_process."log_res", "Variant"=w454) -> (w452:cluster{"Proc":T1, "Variant":variant})  [unwired: 1 in]
        n211 = Enqueue Element(queue=w456, element=w452, error in (no error)=w439) -> ()  [unwired: 1 in, 3 out]
        n212 = property on="testing?" class="Bool (strict)"(error in=w444, "Blinking"=w441) -> (error out=w442:errorcluster)  [unwired: 1 in, 1 out]
        n213 = property on="WL_now" class="DigNum (strict)"(error in=w442, "Visible"=w441) -> ()  [unwired: 1 in, 2 out]
      }
      frame "log_res" {
        n214 = Variant To Data(type=dbl[][] [] ("appended array"), Variant=w499) -> (data=w488:dbl[][])  [unwired: 1 in, 1 out]
        n215 = Transpose 2D Array(2D array=w488) -> (transposed array=w489:dbl[][])
        n216 = local read "Unit(dB:T)"() -> (w484:bool)
        n217 = Number To Fractional String(number=w489, precision (6)=i16 3) -> (F-format string=w487:string[][])  [unwired: 2 in]
        n218 = case shown="False" w484 {
          tunnel: w487 -> [w518 w525]
          tunnel: [w516 w524] -> w483
          tunnel: w485 -> [_ w521]
          frame False {
            n219 = Build Array (concatenate)(string[] ["WL", "IL(dBm)"], w518) -> (w516:string[][])
          }
          frame True {
            n220 = Number To Fractional String(number=w521, precision (6)=i16 3) -> (F-format string=w520:string)  [unwired: 2 in]
            n221 = Build Array (concatenate)(string[] ["WL", "IL(dB)", "", "Ref(dBm)"], w520) -> (w523:string[])
            n222 = Build Array (concatenate)(w523, w525) -> (w524:string[][])
          }
        }
        n223 = case shown="True" "myFname" {
          tunnel: w483 -> [_ w513]
          tunnel: [errorcluster {"status"=TRUE, "code"=0, "source"=""} ("error out") w512] -> w481
          frame False {
          }
          frame True {
            n224 = call-poly <vilib>:"Write Delimited Spreadsheet.vi"("file path (dialog if empty)"=path "", "2D data"=w513, "delimiter (\\t)"="," ("delimiter (\\t)")) -> ("error out"=w512:errorcluster)  [unwired: 11 in, 1 out]
          }
        }
        n225 = case shown="Error" w481 {
          selector: w481 -> [w501 _]
          tunnel: [w501 w508] -> w486
          tunnel: w483 -> [_ w502]
          frame No Error {
          }
          frame Error {
            n226 = Format Date/Time String(time format string (%c)="%m%d%H%M.csv") -> (date/time string=w504:string)  [unwired: 2 in]
            n227 = Concatenate Strings("log_scanpeak_" ("string"), w504) -> (w503:string)
            n228 = call <vilib>:"Application Directory.vi"() -> ("Application Directory"=w507:path)
            n229 = Build Path(base path=w507, name or relative path=w503) -> (appended path=w509:path)
            n230 = call-poly <vilib>:"Write Delimited Spreadsheet.vi"("file path (dialog if empty)"=w509, "2D data"=w502, "delimiter (\\t)"="," ("delimiter (\\t)")) -> ("error out"=w508:errorcluster)  [unwired: 11 in, 1 out]
          }
        }
        n231 = Unbundle By Name(w486) -> ("status"=w497:bool)
        n232 = property on="Msg" class="Str"() -> ("Value"=w494:string)  [unwired: 2 in, 2 out]
        n233 = Select(t="log not saved.", s=w497, f="log saved.") -> (s? t:f=w495:string)
        n234 = Concatenate Strings(w494, w495) -> (w496:string)
        n235 = property on="Msg" class="Str"("Value"=w496) -> ()  [unwired: 2 in, 2 out]
      }
      frame "quit" {
        w527 = FALSE ("link?")
        n236 = Variant To Data(type=FALSE, Variant=w533) -> (data=w531:bool)  [unwired: 1 in, 1 out]
        n237 = case shown="True" w531 {
          tunnel: w538 -> [w540 w546]
          tunnel: w536 -> [w541 w547]
          tunnel: [w541 w547] -> w535
          tunnel: [w540 w546] -> w534
          tunnel: w529 -> [w539 w542]
          tunnel: [w539 w544] -> w528
          frame False {
          }
          frame True {
            n238 = call "OSICS_Closeport.vi"("error in"=w542, "VISA IN"=w546) -> ("error out"=w545:errorcluster)  [unwired: 9 in]
            n239 = call "PM100D_Close.vi"("error in (no error)"=w542, "VISA resource name"=w547) -> ("error out"=w543:errorcluster)  [unwired: 1 in]
            n240 = Merge Errors(w543, w545) -> (w544:errorcluster)
          }
        }
        n241 = property on="link?" class="Bool (strict)"("Value"=w527) -> ()  [unwired: 2 in, 2 out]
        n242 = property on="REF?" class="Bool (strict)"("Value"=w527) -> ()  [unwired: 2 in, 2 out]
        n243 = property on="testing?" class="Bool (strict)"("Blinking"=w527) -> ()  [unwired: 2 in, 2 out]
      }
    }
    "error IO" <- w201
  }
  n244 = Release Queue(queue=w12, error in (no error)=w11) -> ()  [unwired: 1 in, 3 out]
